vi "Get LR700 data_GPIB.vi"(4 "error in (no error)":errorcluster, 5 "Data chanel":enum16{"R", "X"}(ring), 6 "Max repetitions":i32=6, 7 "GPIB Addr":i16) -> (0 "error out":errorcluster, 2 "Data":dbl format="%.4e")   [LabVIEW 2015]
uses:
  GPIB/GPIB Send Receive.vi
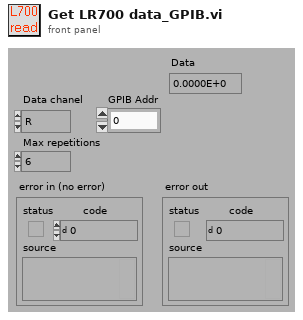
[diagram p1: front panel]
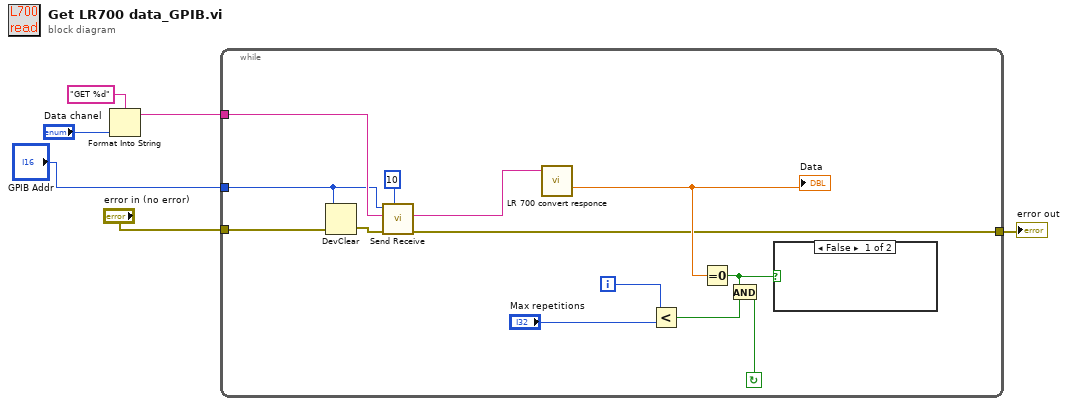
[diagram p0: block diagram]
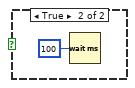
[diagram p2: hidden frame]
diagram:
  n1 = Format Into String(format string="GET %d", "Data chanel") -> (resulting string=w4:string)  [unwired: 2 in, 1 out]
  n2 = while {
    tunnel: [w8] -> w2
    tunnel: "error in (no error)" -> [w9]
    tunnel: w4 -> [w13]
    tunnel: "GPIB Addr" -> [w7]
    i -> [w18]
    stop <- w15 continue-if-true
    n3 = DevClear(2:w9, 4:w7) -> (0:w12:errorcluster)  [unwired: 2 out]
    n4 = call-poly "Send Receive.vi"("Delay, ms"=u32 10, "error in (no error)"=w12, "data string in"=w13, "GPIB Adress"=w7) -> ("error out"=w8:errorcluster, "data string out"=w10:string)  [unwired: 5 in, 1 out]
    n5 = call "LR 700 convert responce.vi"("LR 700 Responce"=w10) -> ("Resistance"=w19:dbl)  [unwired: 2 out]
    "Data" <- w19
    n6 = Less?(x=w18, y="Max repetitions") -> (x < y?=w16:bool)
    n7 = Equal To 0?(x=w19) -> (x = 0?=w14:bool)
    n8 = And(x=w14, y=w16) -> (x .and. y?=w15:bool)
    n9 = case shown="False" w14 {
      frame False {
      }
      frame True {
        n10 = Wait (ms)(milliseconds to wait=u32 100) -> ()  [unwired: 1 out]
      }
    }
  }
  "error out" <- w2
